vi "timerfd_gettime.vi"(8 "error in (no error)":errorcluster, 11 "fd in":i32) -> (0 "error out":errorcluster, 2 "current value":T1, 3 "fd out":i32)   [LabVIEW 2013, in "Linux RT IPC.C.lvlib"]
uses:
  Linux RT IPC.C.lvlib
  Controls/functions.ctl
  <vilib>/NI/NI Linux RT Errno/Linux Errno.lvlib
  <vilib>/NI/NI Linux RT Utilities/Linux RT Utilities.lvlib
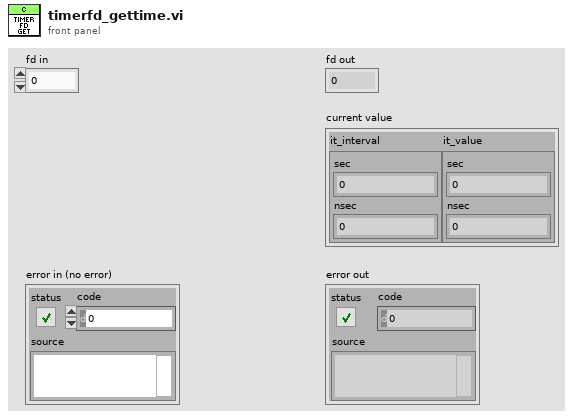
[diagram p1: front panel]
types:
  T1 = cluster{"it_interval":cluster{"sec":u64, "nsec":u64}, "it_value":cluster{"sec":u64, "nsec":u64}}
  T2 = cluster{"it_interval":cluster{"sec":u32, "nsec":u32}, "it_value":cluster{"sec":u32, "nsec":u32}}
  T3 = cluster{"timespec 64":cluster{"sec":u64, "nsec":u64}, "timespec 64":cluster{"sec":u64, "nsec":u64}}
  T4 = typedef "Linux RT IPC.C.lvlib/functions.ctl" = enum16{"unspecified", "close", "epoll_create", "epoll_ctl", "epoll_wait", "fstat", "ftruncate", "mkfifo", "mmap", "munmap", "open", "read", "shm_open", "shm_unlink", "timerfd_create", "timerfd_settime", "timerfd_gettime", "write", "unlink"}
  T5 = typedef "Linux Errno.lvlib/errno.ctl" = enum16{"NO ERROR", "EPERM", "ENOENT", "ESRCH", "EINTR", "EIO", "ENXIO", "E2BIG", "ENOEXEC", "EBADF", "ECHILD", "EAGAIN", "ENOMEM", "EACCES", "EFAULT", "ENOTBLK", "EBUSY", "EEXIST", "EXDEV", "ENODEV", "ENOTDIR", "EISDIR", "EINVAL", "ENFILE", "EMFILE", "ENOTTY", "ETXTBSY", "EFBIG", "ENOSPC", "ESPIPE", "EROFS", "EMLINK", "EPIPE", "EDOM", "ERANGE", "EDADLK", "ENAMETOOLONG", "ENOLCK", "ENOSYS", "ENOTEMPTY", "ELOOP", "EWOULDBLOCK", "ENOMSG", "EIDRM", "ECHRNG", "EL2NSYNC", "EL3HLT", "EL3RST", "ELNRNG", "EUNATCH", "ENOCSI", "EL2HLT", "EBADE", "EBADR", "EXFULL", "ENOANO", "EBADRQC", "EBADSLT", "EDEADLOCK", "EBFONT", "ENOSTR", "ENODATA", "ETIME", "ENOSR", "ENONET", "ENOPKG", "EREMOTE", "ENOLINK", "EADV", "ESRMNT", "ECOMM", "EPROTO", "EMULTIHOP", "EDOTDOT", "EBADMSG", "EOVERFLOW", "ENOTUNIQ", "EBADFD", "EREMCHG", "ELIBACC", "ELIBBAD", "ELIBSCN", "ELIBMAX", "ELIBEXEC", "ELISEQ", "ERESTART", "ESTRPIPE", "EUSERS", "ENOTSOCK", "EDESTADDRREQ", "EMSGSIZE", "EPROTOTYPE", "ENOPROTOOPT", "EPROTONOSUPPORT", "ESOCKTNOSUPPORT", "EOPNOTSUPP", "EPFNOSUPPORT", "EAFNOSUPPORT", "EADDRINUSE", "EADDRNOTAVAIL", "ENETDOWN", "ENETUNREACH", "ENETRESET", "ECONNABORTED", "ECONNRESET", "ENOBUFS", "EISCONN", "ENOTCONN", "ESHUTDOWN", "ETOOMANYREFS", "ETIMEDOUT", "ECONNREFUSED", "EHOSTDOWN", "EHOSTUNREACH", "EALREADY", "EINPROGRESS", "ESTALE", "EUCLEAN", "ENOTNAM", "ENAVAIL", "EISNAM", "EREMOTEIO", "EDQUOT", "ENOMEDIUM", "EMEDIUMTYPE", "ECANCELED", "ENOKEY", "EKEYEXPIRED", "EKEYREVOKED", "EKEYREJECTED", "EOWNERDEAD", "ENOTRECOVERABLE", "ERFKILL", "EHWPOISON", "UNDEFINED"}
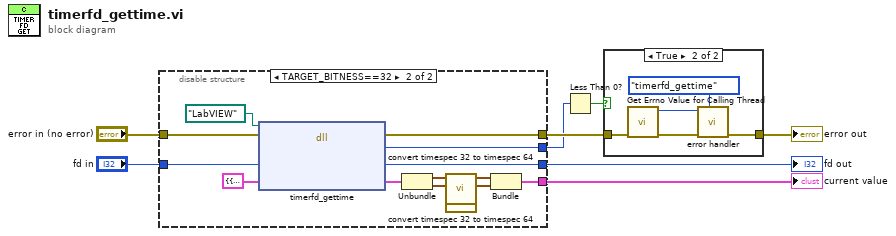
[diagram p0: block diagram]
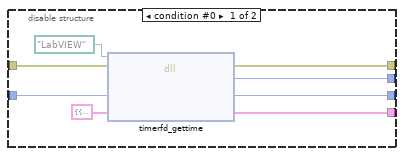
[diagram p2: hidden frame]
diagram:
  n1 = disable-structure shown="TARGET_BITNESS==32" {
    disable-tunnel: "error in (no error)" -> [w16 w29]
    disable-tunnel: [w15 w28] -> w7
    disable-tunnel: [w12 w17] -> w4
    disable-tunnel: [w11 w25] -> w3
    disable-tunnel: "fd in" -> [w10 w24]
    disable-tunnel: [w9 w23] -> w1
    frame condition #0 {
      n2 = dll-call lib="LabVIEW" fn="timerfd_gettime"(path in=path "LabVIEW", error in=w16, "fd"=w10, "curr_value"=T1 {"it_interval"={"sec"=0, "nsec"=0}, "it_value"={"sec"=0, "nsec"=0}} ("old value")) -> (error out=w15:errorcluster, "return"=w9:i32, "fd"=w11:i32, "curr_value"=w12:T1)  [unwired: 1 in, 1 out]
    }
    frame condition #1 (active) {
      n3 = dll-call lib="LabVIEW" fn="timerfd_gettime"(path in=path "LabVIEW", error in=w29, "fd"=w24, "curr_value"=T2 {"it_interval"={"sec"=0, "nsec"=0}, "it_value"={"sec"=0, "nsec"=0}} ("old value")) -> (error out=w28:errorcluster, "return"=w23:i32, "fd"=w25:i32, "curr_value"=w18:T2)  [unwired: 1 in, 1 out]
      n4 = Unbundle(w18) -> ("it_interval"=w19:cluster{"sec":u32, "nsec":u32}, "it_value"=w21:cluster{"sec":u32, "nsec":u32})
      n5 = call <vilib>:"convert timespec 32 to timespec 64.vi"("timespec 32"=w19) -> ("timespec 64"=w20:cluster{"sec":u64, "nsec":u64})  [unwired: 10 in]
      n6 = call <vilib>:"convert timespec 32 to timespec 64.vi"("timespec 32"=w21) -> ("timespec 64"=w22:cluster{"sec":u64, "nsec":u64})  [unwired: 10 in]
      n7 = Bundle("timespec 64"=w20, "timespec 64"=w22) -> (w17:T3)  [unwired: 1 in]
    }
  }
  "fd out" <- w3
  "current value" <- w4
  n8 = Less Than 0?(x=w1) -> (x < 0?=w5:bool)
  n9 = case shown="True" w5 {
    tunnel: w7 -> [w30 w35]
    tunnel: [w30 w34] -> w6
    frame False {
    }
    frame True {
      n10 = call <vilib>:"Get Errno Value for Calling Thread.vi"("error in (no error)"=w35) -> ("error out"=w32:errorcluster, "errno"=w33:T5)  [unwired: 9 in]
      n11 = call "error handler.vi"("function (unspecified)"=functions."timerfd_gettime" ("function"), "error in (no error)"=w32, "errno"=w33) -> ("error out"=w34:errorcluster)  [unwired: 8 in]
    }
  }
  "error out" <- w6
